vi "Get Next Identifier.vi"(8 "error in":errorcluster, 11 "Reset IDs":bool) -> (0 "error out":errorcluster, 3 "ID":u32)   [LabVIEW 2020, in "Ballard ARINC 429 Hardware Configuration.lvlib"]
uses:
  Ballard ARINC 429 Hardware Configuration.lvlib
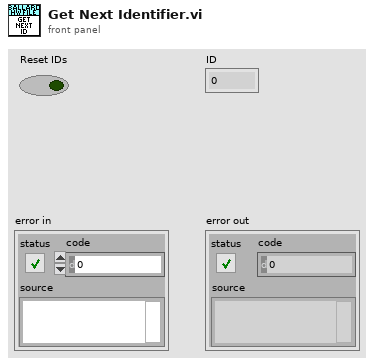
[diagram p1: front panel]
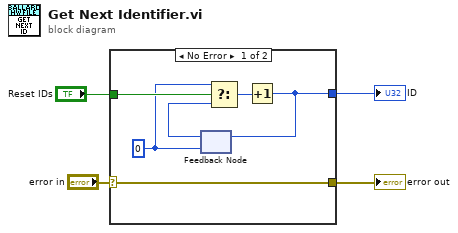
[diagram p0: block diagram]
diagram:
  n1 = case shown="No Error" "error in" {
    selector: "error in" -> [w5 w11]
    tunnel: "Reset IDs" -> [w10 _]
    tunnel: [w6 _] -> w3
    tunnel: [w5 w11] -> w1
    frame No Error {
      w7 = u32 0 ("ID")
      n2 = feedback #1(w7) -> (w8:u32)
      n3 = Select(t=w7, s=w10, f=w8) -> (s? t:f=w9:u32)
      n4 = Increment(x=w9) -> (x+1=w6:u32)
      n5 = feedback-in #1(w6) -> ()
    }
    frame Error {
    }
  }
  "error out" <- w1
  "ID" <- w3
